vi "menu.vi"() -> (0 "s? t:f":T1(ring))   [LabVIEW 2023]
panel:
  in  "odbierz":bool
  in  "zaparkuj":bool
  # "CO CHCESZ?"
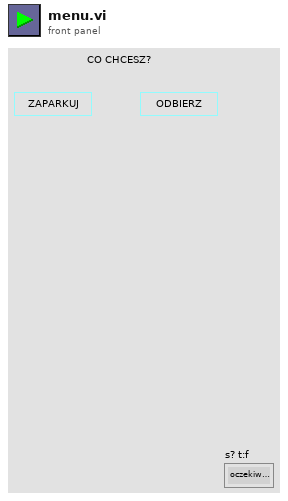
[diagram p1: front panel]
types:
  T1 = enum16{"oczekiwanie", "start", "wpisywanie rejestracji1", "wpisywanie rejestracji2", "zaplata za 1h", "wyjazd z parkingu", "wjazd auta", "doplata"}
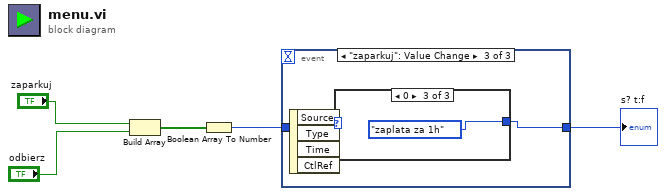
[diagram p0: block diagram]
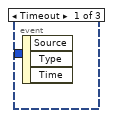
[diagram p2: hidden frame]
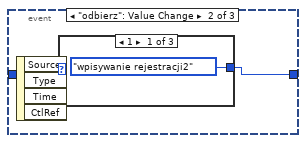
[diagram p3: hidden frame]
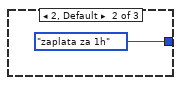
[diagram p4: hidden frame]
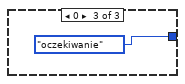
[diagram p5: hidden frame]
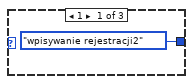
[diagram p6: hidden frame]
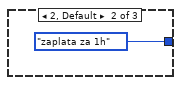
[diagram p7: hidden frame]
diagram:
  n1 = Build Array("zaparkuj", "odbierz") -> (w5:bool[])
  n2 = Boolean Array To Number(Boolean array=w5) -> (number=w4:u32)
  n3 = event shown="[2] \"zaparkuj\": Value Change" {
    selector: _ -> [_ _ _]
    dyn-events: _ -> [_ _ _]
    timeout: _ -> [_ _ _]
    tunnel: w4 -> [_ w7 w12]
    tunnel: [_ w6 w11] -> w3
    event Timeout {
      n4 = event-data() -> ()  [unwired: 1 in, 3 out]
    }
    event "odbierz": Value Change {
      n5 = event-data() -> ()  [unwired: 1 in, 4 out]
      n6 = case shown="1" w7 {
        tunnel: [T1."wpisywanie rejestracji2" T1."zaplata za 1h" T1."oczekiwanie"] -> w6
        frame 1 {
        }
        frame 2, Default {
        }
        frame 0 {
        }
      }
    }
    event "zaparkuj": Value Change {
      n7 = event-data() -> ()  [unwired: 1 in, 4 out]
      n8 = case shown="0" w12 {
        tunnel: [T1."wpisywanie rejestracji2" T1."zaplata za 1h" T1."zaplata za 1h"] -> w11
        frame 1 {
        }
        frame 2, Default {
        }
        frame 0 {
        }
      }
    }
  }
  "s? t:f" <- w3
